vi "ProtocolAnalysis00.vi"(0 "TCP ref in":refnum<k5>, 11 "error in":errorcluster caption="错误输入") -> (3 "AA":string, 4 "TCP ref out":refnum<k5>, 6 "Exit":bool, 8 "string":string, 14 "55":string, 15 "error out":errorcluster caption="错误输出")   [LabVIEW 2014]
uses:
  DataBase/DataBase.lvlib
panel:
  out "计数":i32
  out "长度":u8
  out "x = y?":bool
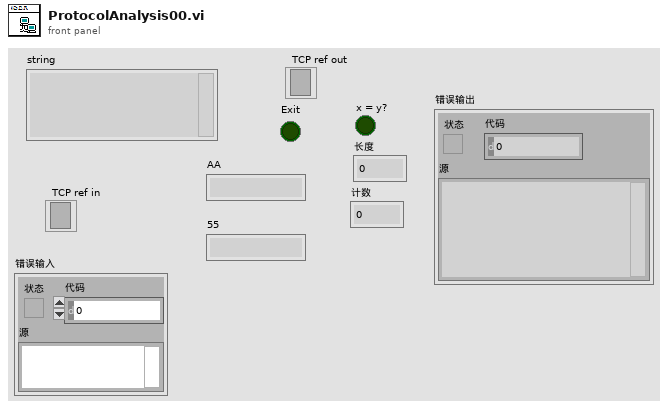
[diagram p1: front panel]
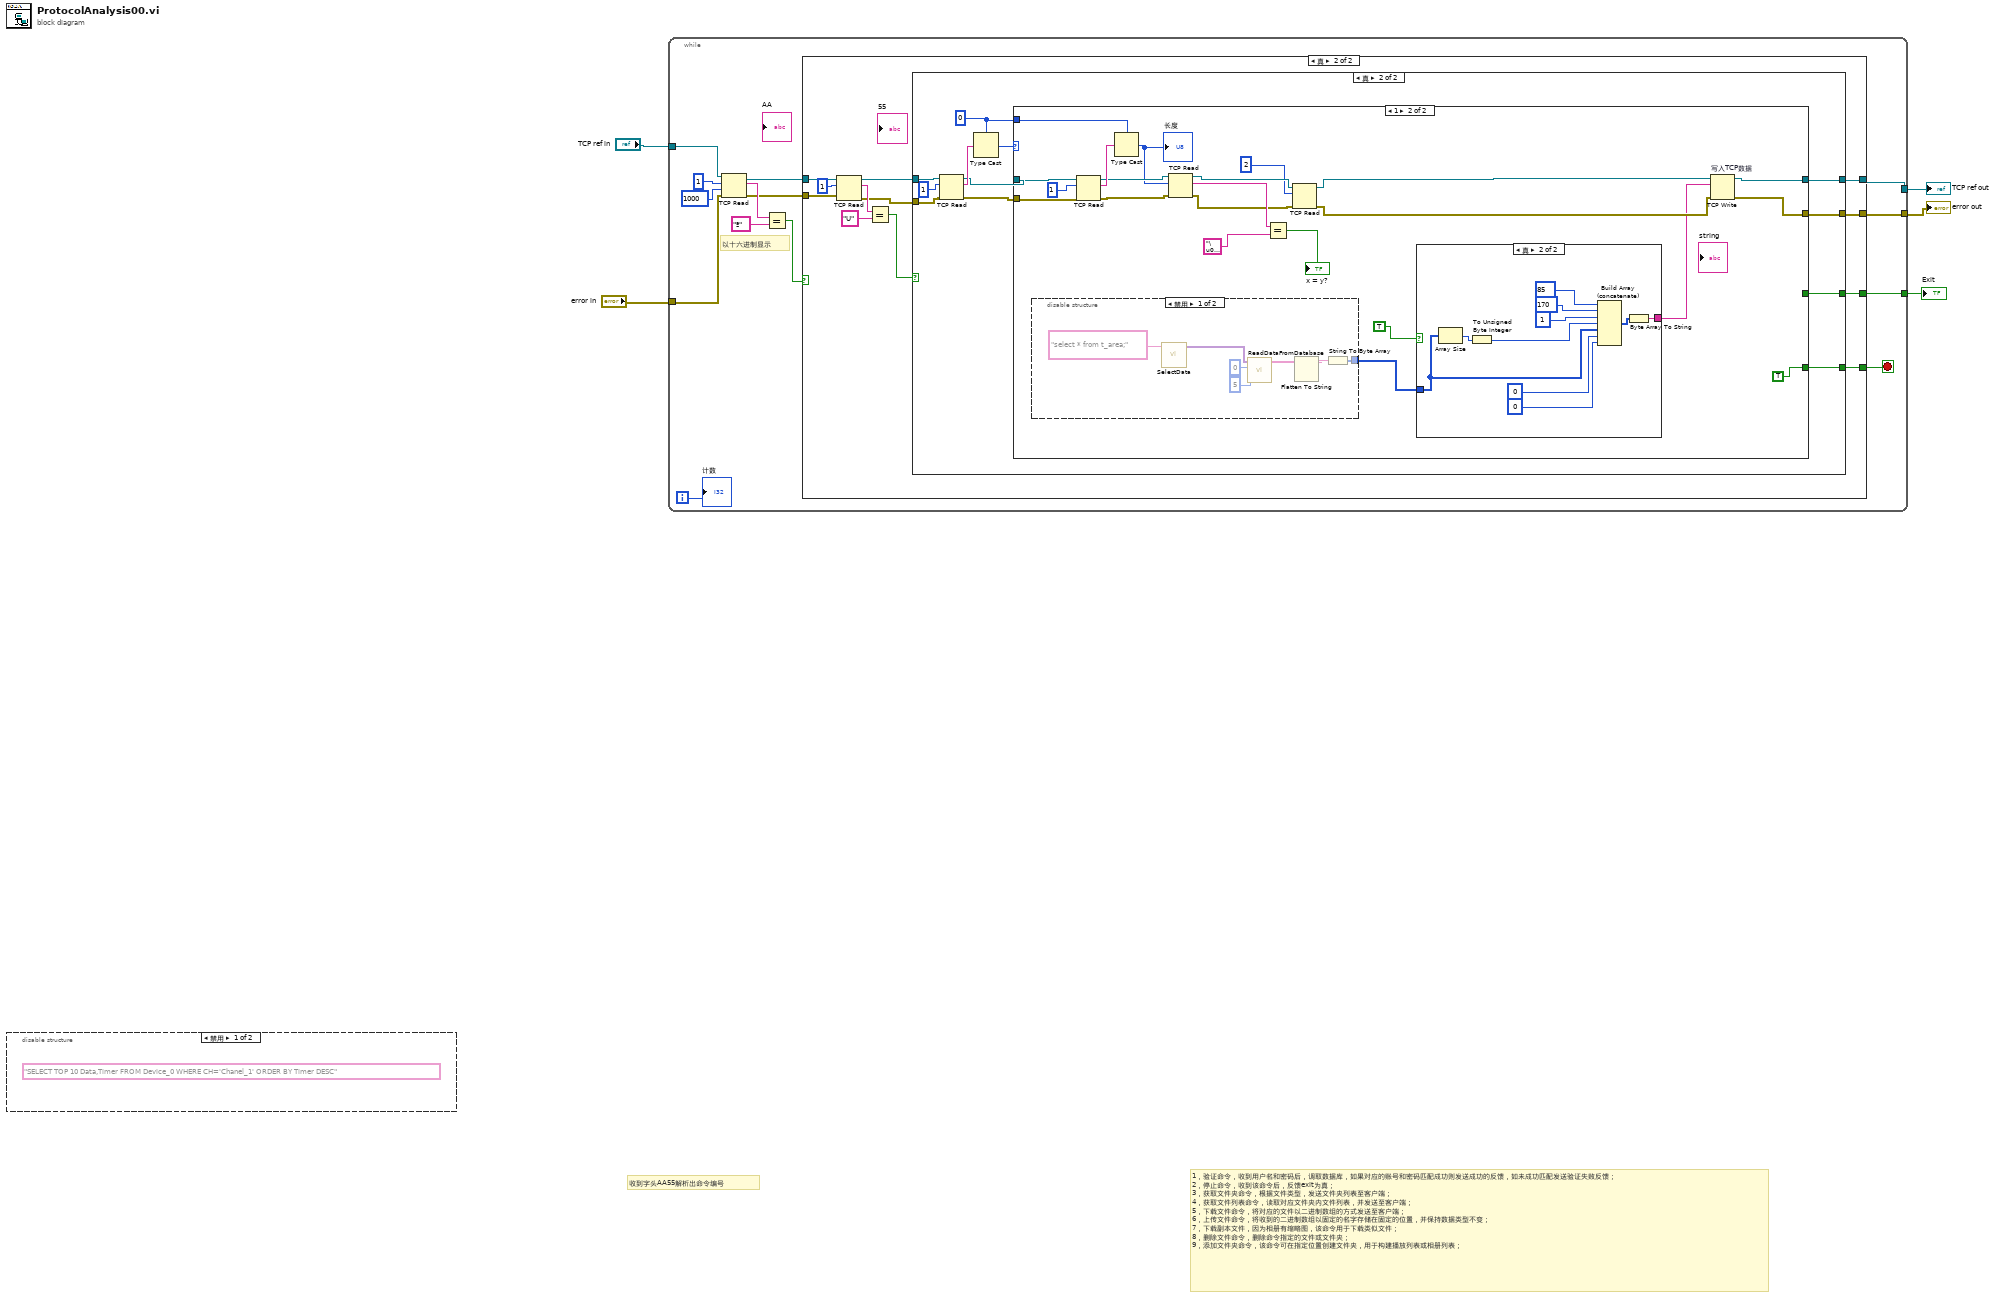
[diagram p0: block diagram]
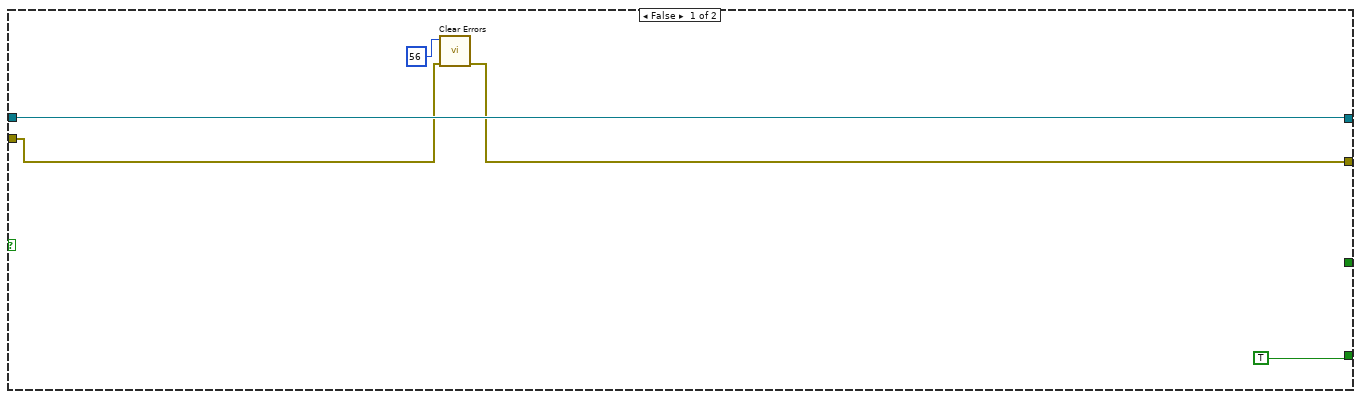
[diagram p2: hidden frame]
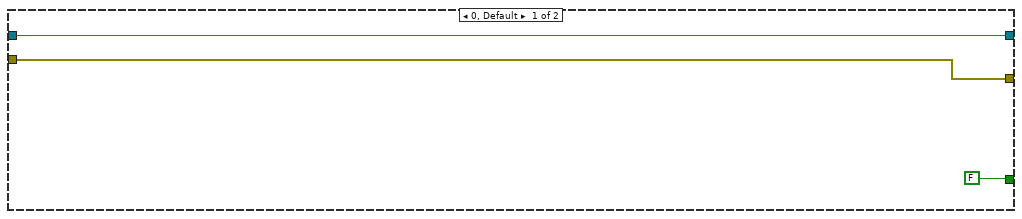
[diagram p4: hidden frame]
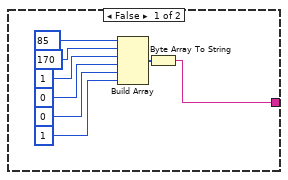
[diagram p6: hidden frame]
diagram:
  # "1，验证命令，收到用户名和密码后，调取数据库，如果对应的账号和密码匹配成功则发送成功的反馈，如未成功匹配发送验证失败反馈；\n2，停止命令，收到该命令后，反馈exit为真；\n3，获取文件夹命令，根据文件类型，发送文件夹列表至客户端；\n4，获取文件列表命令，读取对应文件夹内文件列表，并发送至客户端；\n5，下载文件命令，将对应的文件以二进制数组的方式发送至客户端；\n6，上传文件命令，将收到的二进制数组以固定的名字存储在固定的位置，并保持数据类型不变；\n7，下载副本文件，因为相册有缩略图，该命令用于下载类似文件；\n8，删除文件命令，删除命令指定的文件或文件夹；\n9，添加文件夹命令，该命令可在指定位置创建文件夹，用于构建播放列表或相册列表；"
  # "收到字头AA55解析出命令编号"
  n1 = disable-structure shown="禁用" {
    frame Disabled {
      (unwired) "SELECT TOP 10 Data,Timer FROM Device_0 WHERE CH='Chanel_1' ORDER BY Timer DESC" ("SQL query")
    }
    frame Enabled {
    }
  }
  n2 = while {
    tunnel: "TCP ref in" -> [w19]
    tunnel: "error in" -> [w18]
    tunnel: [w10] -> w3
    tunnel: [w9] -> w2
    tunnel: [w7] -> w1
    i -> [w6]
    stop <- w8 stop-if-true
    # "以十六进制显示"
    n3 = TCP Read(connection ID=w19, bytes to read=1 ("读取的字节"), error in (no error)=w18, 9:1000 ("超时毫秒(25000)")) -> (connection ID out=w12:refnum<k5>, data out=w15:string, error out=w11:errorcluster)  [unwired: 1 in]
    n4 = Equal?(x=w15, y="ª") -> (x = y?=w13:bool)
    n5 = case shown="真" w13 {
      tunnel: w12 -> [w24 w33]
      tunnel: w11 -> [w22 w32]
      tunnel: [w24 w28] -> w10
      tunnel: [w21 w27] -> w9
      tunnel: [TRUE w26] -> w8
      tunnel: [_ w25] -> w7
      frame False {
        n6 = call <vilib>:"Clear Errors.vi"("error in (no error)"=w22, "specific error code to clear (0: all)"=56) -> ("error out"=w21:errorcluster)  [unwired: 4 in, 1 out]
      }
      frame True {
        n7 = TCP Read(connection ID=w33, bytes to read=1 ("读取的字节"), error in (no error)=w32) -> (connection ID out=w29:refnum<k5>, data out=w35:string, error out=w30:errorcluster)  [unwired: 2 in]
        n8 = Equal?(x=w35, y="U") -> (x = y?=w31:bool)
        n9 = case shown="真" w31 {
          tunnel: w30 -> [w37 w48]
          tunnel: w29 -> [w38 w47]
          tunnel: [w38 w44] -> w28
          tunnel: [w37 w43] -> w27
          tunnel: [_ w41] -> w26
          tunnel: [_ w39] -> w25
          frame False {
          }
          frame True {
            w40 = u8 0
            n10 = TCP Read(connection ID=w47, bytes to read=1 ("读取的字节"), error in (no error)=w48) -> (connection ID out=w45:refnum<k5>, data out=w49:string, error out=w42:errorcluster)  [unwired: 2 in]
            n11 = Type Cast(type=w40, x=w49) -> (*(type *) &x=w46:u8)
            n12 = case shown="1" w46 {
              tunnel: w45 -> [w53 w71]
              tunnel: [w53 w75] -> w44
              tunnel: [w52 w74] -> w43
              tunnel: w42 -> [w52 w70]
              tunnel: [_ TRUE] -> w41
              tunnel: w40 -> [_ w69]
              tunnel: [FALSE _] -> w39
              frame 0, Default {
              }
              frame 1 {
                n13 = disable-structure shown="禁用" {
                  disable-tunnel: [w76 _] -> w56
                  frame Disabled {
                    n14 = call "SelectData.vi"("SQL query"="select * from t_area;") -> ("recordset data"=w81:variant[][])  [unwired: 7 in, 1 out]
                    n15 = call "ReadDataFromDatabase.vi"("长度"=5, "index"=0, "recordset data"=w81) -> ("所有记录"=w77:string[][])  [unwired: 7 in, 1 out]
                    n16 = Flatten To String(anything=w77) -> (data string=w78:string)  [unwired: 3 in, 2 out]
                    n17 = String To Byte Array(string=w78) -> (unsigned byte array=w76:u8[])
                  }
                  frame Enabled {
                  }
                }
                n18 = TCP Read(connection ID=w71, bytes to read=1 ("读取的字节"), error in (no error)=w70) -> (connection ID out=w67:refnum<k5>, data out=w68:string, error out=w60:errorcluster)  [unwired: 2 in]
                n19 = Type Cast(type=w69, x=w68) -> (*(type *) &x=w66:u8)
                "长度" <- w66
                n20 = TCP Read(connection ID=w67, bytes to read=w66, error in (no error)=w60) -> (connection ID out=w62:refnum<k5>, data out=w65:string, error out=w59:errorcluster)  [unwired: 2 in]
                n21 = Equal?(x=w65, y="\u0000") -> (x = y?=→"x = y?":bool)
                n22 = TCP Read(connection ID=w62, bytes to read=2, error in (no error)=w59) -> (connection ID out=w61:refnum<k5>, error out=w58:errorcluster)  [unwired: 2 in, 1 out]
                n23 = case shown="真" TRUE {
                  tunnel: w56 -> [_ w94]
                  tunnel: [w83 w93] -> w55
                  frame False {
                    n24 = Build Array(u8 85, u8 170, u8 1, u8 0, u8 0, u8 1) -> (w84:u8[])
                    n25 = Byte Array To String(unsigned byte array=w84) -> (string=w83:string)
                  }
                  frame True {
                    n26 = Array Size(array=w94) -> (size(s)=w96:i32)
                    n27 = To Unsigned Byte Integer(number=w96) -> (unsigned 8bit integer=w95:u8)
                    n28 = Build Array (concatenate)(u8 85, u8 170, u8 1, w95, w94, u8 0, u8 0) -> (w97:u8[])
                    n29 = Byte Array To String(unsigned byte array=w97) -> (string=w93:string)
                  }
                }
                n30 = TCP Write "写入TCP数据"(connection ID=w61, data in=w55, error in (no error)=w58) -> (connection ID out=w75:refnum<k5>, error out=w74:errorcluster)  [unwired: 1 in, 1 out]
              }
            }
          }
        }
      }
    }
    "计数" <- w6
  }
  "error out" <- w2
  "TCP ref out" <- w3
  "Exit" <- w1
